vi "Stopwatch FGV.vi"(7 "Stopwatch Action":T1, 8 "Error In":errorcluster) -> (0 "Error Out":errorcluster, 1 "Paused?":bool, 2 "Elapsed Time":dbl)   [LabVIEW 2010]
uses:
  Stopwatch Action.ctl
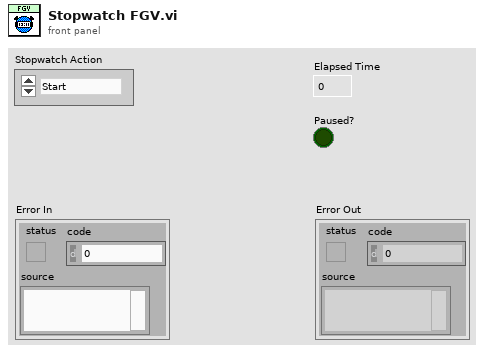
[diagram p1: front panel]
types:
  T1 = typedef "Stopwatch Action.ctl" = enum16{"Start", "Current Time", "Pause", "Reset"}
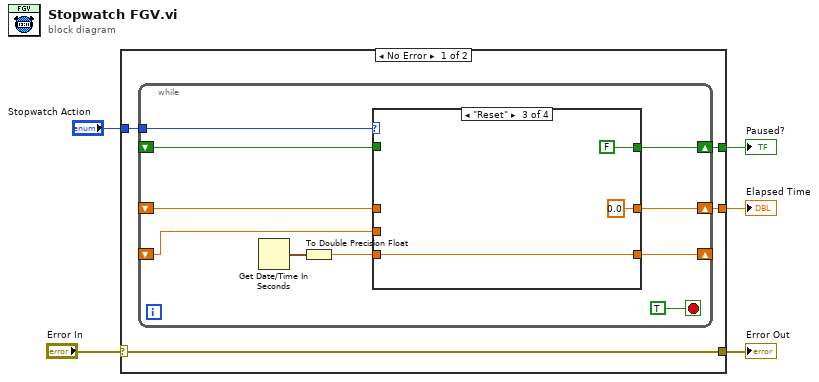
[diagram p0: block diagram]
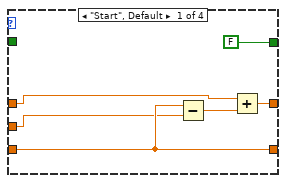
[diagram p2: hidden frame]
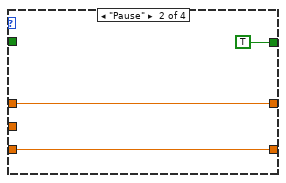
[diagram p3: hidden frame]
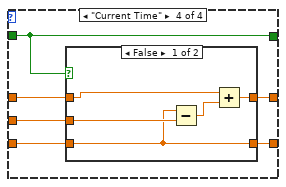
[diagram p4: hidden frame]
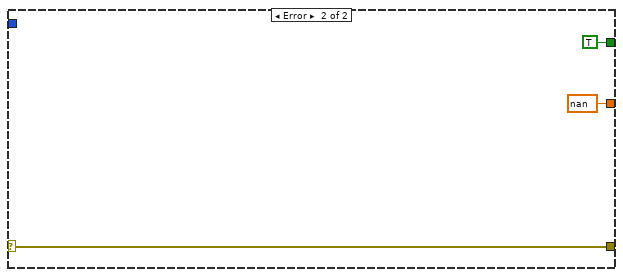
[diagram p6: hidden frame]
diagram:
  n1 = case shown="No Error" "Error In" {
    selector: "Error In" -> [w6 w47]
    tunnel: [w9 TRUE] -> w5
    tunnel: [w8 nan] -> w4
    tunnel: "Stopwatch Action" -> [w7 _]
    tunnel: [w6 w47] -> w1
    frame No Error {
      n2 = while {
        shift-right: [w19] -> w8
        shift-left: _ -> [w16]
        shift-right: [w18] -> _
        shift-left: _ -> [w17]
        shift-right: [w13] -> w9
        shift-left: _ -> [w11]
        tunnel: w7 -> [w10]
        stop <- TRUE stop-if-true
        n3 = Get Date/Time In Seconds() -> (seconds since 1Jan1904=w15:timestamp)
        n4 = To Double Precision Float(number=w15) -> (double precision float=w14:dbl)
        n5 = case shown="\"Reset\"" w10 {
          tunnel: [w22 w26 0.0 w35] -> w19
          tunnel: w16 -> [w20 w26 _ w36]
          tunnel: [w24 w27 w30 w34] -> w18
          tunnel: [FALSE TRUE FALSE w37] -> w13
          tunnel: w11 -> [_ _ _ w37]
          tunnel: w17 -> [w23 _ _ w33]
          tunnel: w14 -> [w24 w27 w30 w32]
          frame "Start", Default {
            n6 = Subtract(x=w24, y=w23) -> (x-y=w21:dbl)
            n7 = Add(x=w20, y=w21) -> (x+y=w22:dbl)
          }
          frame "Pause" {
          }
          frame "Reset" {
          }
          frame "Current Time" {
            n8 = case shown="False" w37 {
              tunnel: [w42 w44] -> w35
              tunnel: w36 -> [w38 w44]
              tunnel: [w39 w43] -> w34
              tunnel: w33 -> [w40 _]
              tunnel: w32 -> [w39 w43]
              frame False {
                n9 = Subtract(x=w39, y=w40) -> (x-y=w41:dbl)
                n10 = Add(x=w38, y=w41) -> (x+y=w42:dbl)
              }
              frame True {
              }
            }
          }
        }
      }
    }
    frame Error {
    }
  }
  "Paused?" <- w5
  "Elapsed Time" <- w4
  "Error Out" <- w1
